vi "LVCAM Destroy.vi"(10 "Error":errorcluster, 11 "Actor in":refnum<class "Actor.lvclass">) -> ()   [LabVIEW 2021, in "LVCAM.lvlib" / "Actor.lvclass"]
uses:
  Actor.lvclass
  C:/PPLs/LabVIEW-Composed-Actor-Model-LVCAM/LabVIEW-Composed-Actor-Model-LVCAM/LVCAM/LVCAM/LVCAM/LVCAM.lvclass
  Msgs/LVCAM Nest Destroyed/LVCAM Nest Destroyed Msg/LVCAM Nest Destroyed Msg.lvclass
  C:/PPLs/LabVIEW-Composed-Actor-Model-LVCAM/LabVIEW-Composed-Actor-Model-LVCAM/LVCAM/LVCAM/Msg/Msg.lvclass
  Call Msg Send.vi
  C:/PPLs/LabVIEW-Composed-Actor-Model-LVCAM/LabVIEW-Composed-Actor-Model-LVCAM/LVCAM/Msgs/LVCAM Create Nest/LVCAM Create Nest/LVCAM Create Nest.lvclass
  C:/PPLs/LabVIEW-Composed-Actor-Model-LVCAM/LabVIEW-Composed-Actor-Model-LVCAM/LVCAM/Msgs/LVCAM Destroy Self/LVCAM Destroy Self/LVCAM Destroy Self.lvclass
  C:/PPLs/LabVIEW-Composed-Actor-Model-LVCAM/LabVIEW-Composed-Actor-Model-LVCAM/LVCAM/Msgs/LVCAM Nest Destroyed/LVCAM Nest Destroyed/LVCAM Nest Destroyed.lvclass
  C:/PPLs/LabVIEW-Composed-Actor-Model-LVCAM/LabVIEW-Composed-Actor-Model-LVCAM/LVCAM/LVCAM/LVCAM Create/LVCAM Create.lvclass
  C:/PPLs/LabVIEW-Composed-Actor-Model-LVCAM/LabVIEW-Composed-Actor-Model-LVCAM/LVCAM/LVCAM/LVCAM Destroy/LVCAM Destroy.lvclass
  C:/PPLs/LabVIEW-Composed-Actor-Model-LVCAM/LabVIEW-Composed-Actor-Model-LVCAM/LVCAM/LVCAM/LVCAM Error/LVCAM Error.lvclass
  C:/PPLs/LabVIEW-Composed-Actor-Model-LVCAM/LabVIEW-Composed-Actor-Model-LVCAM/LVCAM/LVCAM/LVCAM Receive/LVCAM Receive.lvclass
  C:/PPLs/LabVIEW-Composed-Actor-Model-LVCAM/LabVIEW-Composed-Actor-Model-LVCAM/LVCAM/LVCAM/Actor/Actor.lvclass
  C:/PPLs/LabVIEW-Composed-Actor-Model-LVCAM/LabVIEW-Composed-Actor-Model-LVCAM/LVCAM/Msgs/LVCAM Nest Destroyed/LVCAM Nest Destroyed Msg/LVCAM Nest Destroyed Msg.lvclass
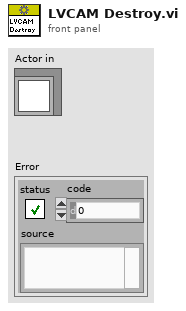
[diagram p1: front panel]
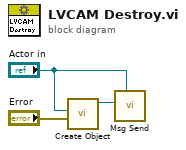
[diagram p0: block diagram]
diagram:
  n1 = call "Create Object.vi"("Nest Error"="Error", "Nest Actor"="Actor in") -> ("LVCAM Nest Destroyed Msg out"=w3:refnum<class "LVCAM Nest Destroyed Msg.lvclass">)  [unwired: 9 in]
  n2 = call-poly "Msg Send.vi"("Actor"="Actor in", "Msg"=w3) -> ()  [unwired: 9 in, 1 out]
